vi "Mover4_ikine_Analytical.vi"() -> ()   [LabVIEW 2015]
uses:
  <vilib>/silver_ctls/ArrayMatrixCluster/Real Matrix NI_Silver.ctl
  <vilib>/robotics/Kinematics/Analytical/6R/Type 1/Analytical Inverse Kinematics (6R Type 1).vi
  <vilib>/robotics/Kinematics/Robot/Forward Kinematics (Point).vi
  <vilib>/robotics/Kinematics/Plotting/NI_Robotics_3DKinematics.lvlib
  <vilib>/robotics/Kinematics/NI_Kinematics.lvlib
  <vilib>/robotics/Kinematics/Analytical/NI_Robotics_AnalyticKinematics.lvlib
  <vilib>/robotics/Kinematics/Analytical/6R/Type 1/NI_Robotics_6R Type 1 Serial Arm Class.lvclass
panel:
  out "end effector transform":T1
  out "Number of valid solutions":i32=8
  out "joint positions":T1=[[-2.356194487692345, -1.9273271474581384, -3.891879829272226, -0.000346143081752452, 2.6775437705794194, 2.356504084119319], [-2.356194487692345, -1.9273271474581384, -3.891879829272226, 3.141246510508041, -2.6775437705794194, -0.7858013974917988], [-2.356194487692345, 1.9219053917026094, 0.9496244806647565, -0.006128043988051504, 0.2699971629553193, 2.350288509844115], [-2.356194487692345, 1.9219053917026094, 0.9496244806647565, 3.135464609601742, -0.2699971629553193, -0.7917289502545055], [0.785398165897448, 1.2188916474893081, -3.8918812175281468, -3.1384124243918667, 0.46853479904264145, 2.3597511429409126], [0.785398165897448, 1.2188916474893081, -3.8918812175281468, 0.003180229197926432, -0.46853479904264145, -0.7825607204386644], [0.785398165897448, -1.215062536550417, 0.9496258689206774, 3.141429516458643, 2.8760853432324827, 2.3567697651301938], [0.785398165897448, -1.215062536550417, 0.9496258689206774, -0.0001631371311500469, -2.8760853432324827, -0.7852407989897241]]
  in  "Desired Analytical solution":i32=2
  in  "z (m)":dbl(slide)=0.2 min=-0.4 max=0.4 step=0.01 scale=0.0..0.5
  in  "y (m)":dbl(slide)=0.1 min=-0.4 max=0.4 step=0.01 scale=-0.4..0.4
  in  "x (m)":dbl(slide)=0.1 min=-0.4 max=0.4 step=0.01 scale=-0.4..0.4
  in  "stop":bool
  out "3D Picture":refnum<vi>(3d-picture)
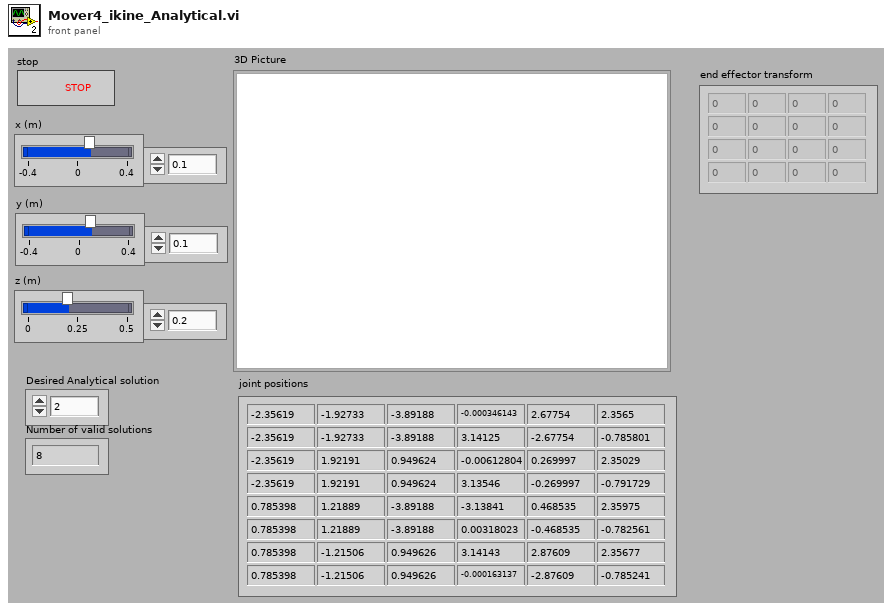
[diagram p1: front panel]
types:
  T1 = typedef "Real Matrix NI_Silver.ctl" = dbl[][]
  T2 = typedef "NI_Matrix.lvlib/RealMatrix.ctl" = dbl[][]
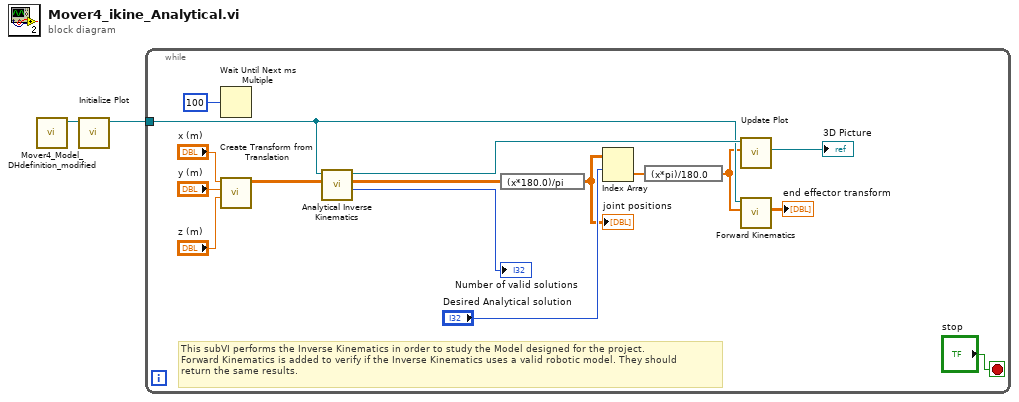
[diagram p0: block diagram]
diagram:
  n1 = call "Mover4_Model_DHdefinition_modified.vi"() -> ("serial arm out"=w1:refnum<class "NI_Robotics_6R Type 1 Serial Arm Class.lvclass">)  [unwired: 10 in, 1 out]
  n2 = call <vilib>:"Initialize Plot.vi"("serial arm in"=w1) -> ("serial arm out"=w2:refnum<class "NI_Robotics_6R Type 1 Serial Arm Class.lvclass">)  [unwired: 9 in, 1 out]
  n3 = while {
    tunnel: w2 -> [w8]
    stop <- "stop" stop-if-true
    # "This subVI performs the Inverse Kinematics in order to study the Model designed for the project.\nForward Kinematics is added to verify if the Inverse Kinematics uses a valid robotic model. They should\nreturn the same results."
    n4 = Wait Until Next ms Multiple(millisecond multiple=u32 100) -> ()  [unwired: 1 out]
    n5 = call <vilib>:"Create Transform from Translation.vi"("z"="z (m)", "y"="y (m)", "x"="x (m)") -> ("transform"=w13:T2)  [unwired: 8 in]
    n6 = call-poly <vilib>:"Analytical Inverse Kinematics.vi"("end effector transform"=w13, "6R type 1 serial arm in"=w8) -> ("number of valid solutions"=→"Number of valid solutions":i32, "joint positions"=w10:T2, "6R type 1 serial arm out"=w16:refnum<class "NI_Robotics_6R Type 1 Serial Arm Class.lvclass">)  [unwired: 6 in, 1 out]
    n7 = expression code="(x*180.0)/pi"(w10) -> (w9:T2)
    "joint positions" <- w9
    n8 = Index Array(array=w9, index (row)="Desired Analytical solution") -> (element=w6:dbl[])  [unwired: 1 in]
    n9 = expression code="(x*pi)/180.0"(w6) -> (w3:dbl[])
    n10 = call <vilib>:"Update Plot.vi"("joint positions"=w3, "serial arm in"=w16) -> ("serial arm scene"=→"3D Picture":refnum<vi>)  [unwired: 7 in, 2 out]
    n11 = call-poly <vilib>:"Forward Kinematics.vi"("joint positions"=w3, "serial arm in"=w8) -> ("end effector transform"=→"end effector transform":T2)  [unwired: 7 in, 2 out]
  }
